vi "FGV-GEvt Filter Obj(lvlibp).vi"(6 "Set? (T)/Get(F)":bool, 8 "Error In":errorcluster caption="error in (no error)", 11 "Rules-v1":T1) -> (0 "error out":errorcluster, 3 "CSM:LogFilter.lvclass":refnum<class "LogFilter.lvclass">)   [LabVIEW 2017, in "Communicable State Machine.lvlib"]
doc: "-- <b>Controls</b> --\n- <b>Set(T)/Get(F)</b>:\n- <b>Rules-v1</b>:\n\n-- <b>Indicators</b> --\n- <b>CSM:LogFilter.lvclass</b>:"
uses:
  Communicable State Machine.lvlib
  LogFilter/LogFilter.lvclass
  Typedef/_CSM_GlobalLog Filter Rules - v1.0.ctl
  Typedef/_CSM_GlobalLog_MSG_TYPE.ctl
  Typedef/_CSM_GlobalLog_STATE_TYPE.ctl
  FGV-GEvt Filter Obj.vi
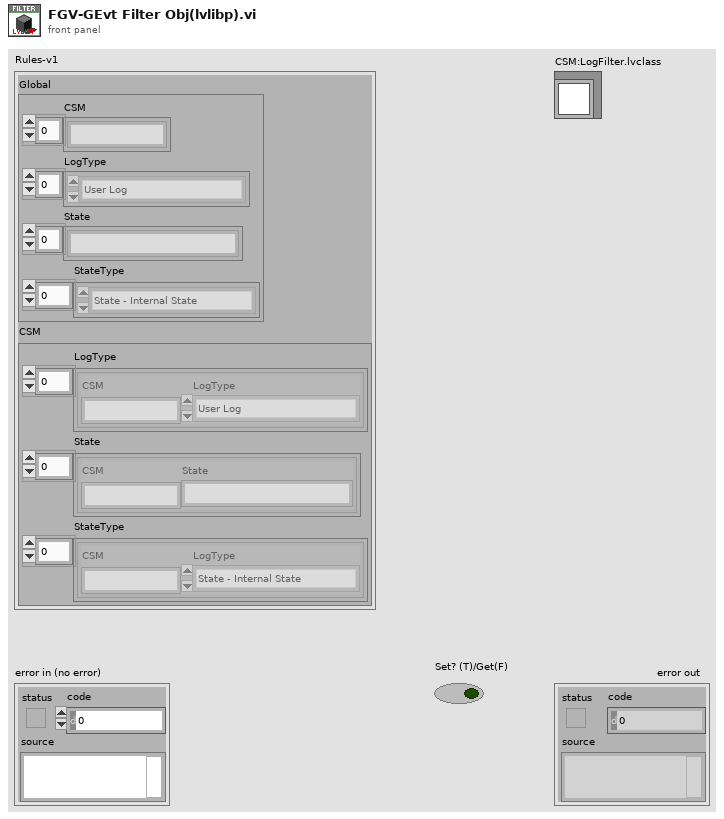
[diagram p1: front panel]
types:
  T1 = typedef "Communicable State Machine.lvlib/_CSM_GlobalLog Filter Rules - v1.0.ctl" = cluster{"Global":cluster{"CSM":string[], "LogType":T2[], "State":string[], "StateType":T3[]}, "CSM":cluster{"LogType":cluster{"CSM":string, "LogType":T2}[], "State":cluster{"CSM":string, "State":string}[], "StateType":cluster{"CSM":string, "LogType":T3}[]}}
  T2 = typedef "Communicable State Machine.lvlib/_CSM_GlobalLog_MSG_TYPE.ctl" = enum16{"User Log", "State Change", "Status", "Interrupt", "Register", "Unregister", "Error Log", "Module Created", "Module Destroyed"}
  T3 = typedef "Communicable State Machine.lvlib/_CSM_GlobalLog_STATE_TYPE.ctl" = enum16{"State - Internal State", "State - External Message", "State - Response", "State - Complete"}
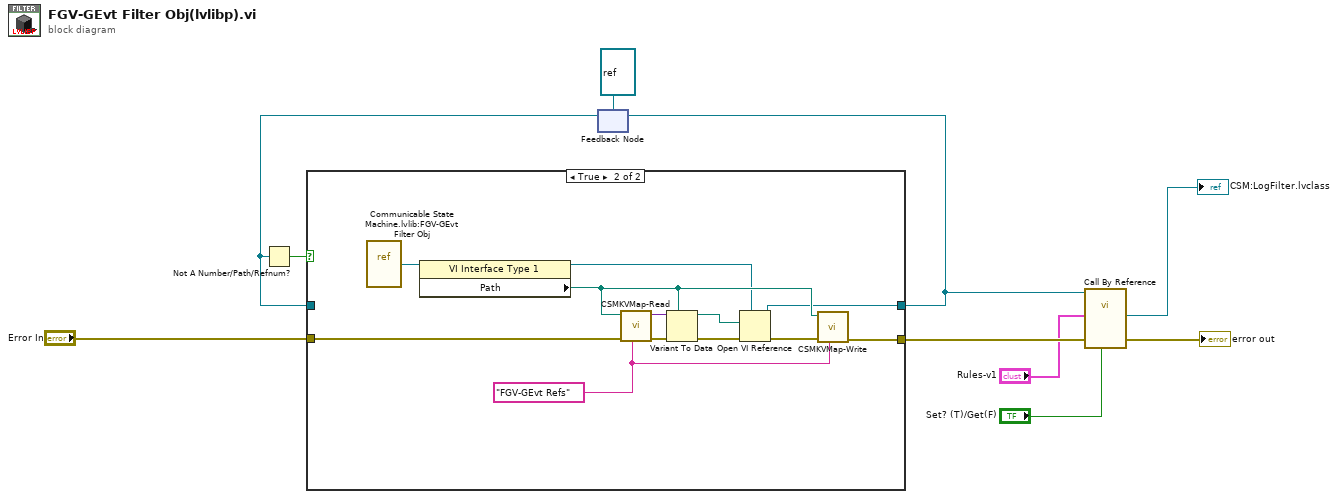
[diagram p0: block diagram]
diagram:
  n1 = feedback #1(refnum<vi> refnum) -> (w9:refnum<vi>)
  n2 = Not A Number/Path/Refnum?(number/path/refnum=w9) -> (NaN/Path/Refnum?=w10:bool)
  n3 = case shown="True" w10 {
    tunnel: [w11 w17] -> w8
    tunnel: [w12 w15] -> w7
    tunnel: "Error In" -> [w12 w14]
    tunnel: w9 -> [w11 _]
    frame False {
    }
    frame True {
      w19 = "FGV-GEvt Refs" ("name")
      n4 = vi-ref "Communicable State Machine.lvlib:FGV-GEvt Filter Obj.vi"() -> (w13:refnum<vi>)
      n5 = property class="VI Interface Type 1"(reference=w13) -> (reference out=w16:refnum<vi>, "Path"=w18:path)  [unwired: 1 in, 1 out]
      n6 = call "CSMKVMap-Read.vi"("name"=w19, "Error in"=w14, "default value (empty variant)"=w18) -> ("Error out"=w24:errorcluster, "value"=w23:variant)  [unwired: 5 in]
      n7 = Variant To Data(error in=w24, type=w18, Variant=w23) -> (data=w22:path, error out=w21:errorcluster)
      n8 = Open VI Reference(type specifier VI Refnum (for type only)=w16, vi path=w22, error in (no error)=w21) -> (vi reference=w17:refnum<vi>, error out=w20:errorcluster)  [unwired: 3 in]
      n9 = call "CSMKVMap-Write.vi"("name"=w19, "Error in"=w20, "value"=w18) -> ("Error out"=w15:errorcluster)  [unwired: 6 in]
    }
  }
  n10 = feedback-in #1(w8) -> ()
  n11 = call-by-ref "?"(reference=w8, "Set? (T)/Get(F)"="Set? (T)/Get(F)", "Error In"=w7, "Rules-v1"="Rules-v1") -> ("error out"=→"error out":errorcluster, "CSM:LogFilter.lvclass"=→"CSM:LogFilter.lvclass":refnum<class "LogFilter.lvclass">)  [unwired: 8 in, 2 out]
